vi "Joystickfunctionfull R (SubVI).vi"   [LabVIEW 2012]
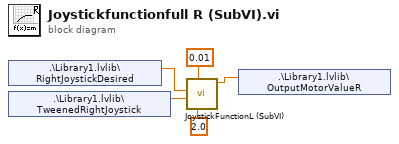
[diagram p0: block diagram]
diagram:
  n1 = shared-variable ".\\Library1.lvlib\\RightJoystickDesired"() -> (w2:dbl)  [unwired: 1 in, 1 out]
  n2 = shared-variable ".\\Library1.lvlib\\TweenedRightJoystick"() -> (w1:dbl)  [unwired: 1 in, 1 out]
  n3 = call "JoystickFunctionL (SubVI).vi"("TimeToReachSpeed"=2.0 ("y"), "DeltaT"=0.01 ("y"), "TweenedSpeed"=w1, "DesiredSpeed"=w2) -> ("OutputMotorValueL"=w3:dbl)  [unwired: 7 in]
  n4 = shared-variable ".\\Library1.lvlib\\OutputMotorValueR"(w3) -> ()  [unwired: 1 in, 1 out]
